vi "Configure Bus Definition.vi"   [LabVIEW 2023, in "Keysight-DSQx3014T.lvlib"]
doc: "Configures bus definition."
uses:
  Keysight-DSQx3014T.lvlib
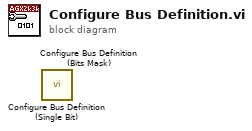
[diagram p0: block diagram]
diagram:
  n1 = call "Configure Bus Definition (Single Bit).vi"() -> ()  [unwired: 10 in, 2 out]
  n2 = call "Configure Bus Definition (Bits Mask).vi"() -> ()  [unwired: 10 in, 2 out]
